vi "Write To Log (append).vi"(8 "Error In":errorcluster, 11 "Text to write":string) -> (0 "Error Out":errorcluster)   [LabVIEW 2023, in "Error Manager.lvlib" / "Error Log.lvclass"]
uses:
  Error Log.lvclass
  Error Log Ref (class variable).vi
  Error Log.lvclass/Error Log.ctl
panel:
  # "Input\nInputs to the VI"
  # "Development\nControls or indicators that are useful for development or testing, but which are not outputs of the VI."
  # "Output\nOutputs of the VI"
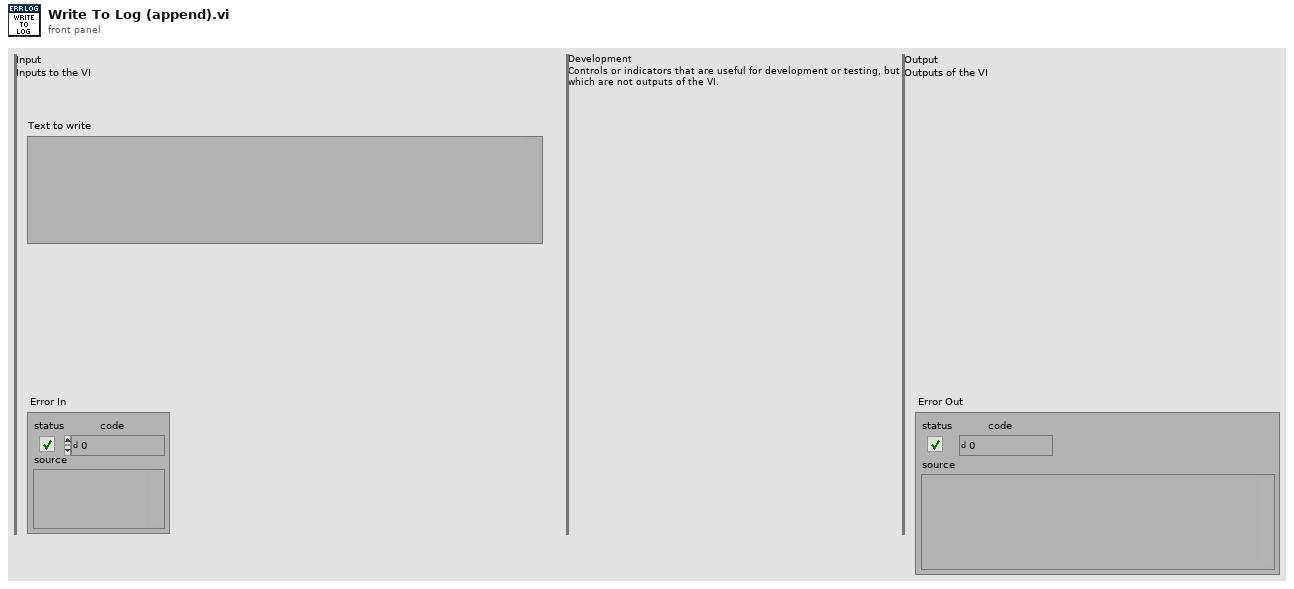
[diagram p1: front panel]
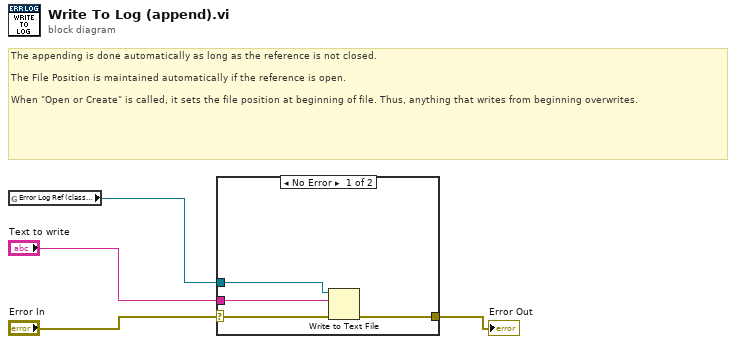
[diagram p0: block diagram]
diagram:
  # "The appending is done automatically as long as the reference is not closed.\n\nThe File Position is maintained automatically if the reference is open.\n\nWhen \"Open or Create\" is called, it sets the file position at beginning of file. Thus, anything that writes from beginning overwrites."
  n1 = global read "Error Log Ref (class variable).vi" item#0() -> (w2:refnum<file>)
  n2 = case shown="No Error" "Error In" {
    selector: "Error In" -> [w8 w9]
    tunnel: "Text to write" -> [w7 _]
    tunnel: w2 -> [w6 _]
    tunnel: [w5 w9] -> w1
    frame No Error {
      n3 = Write to Text File(file (use dialog)=w6, text=w7, error in=w8) -> (error out=w5:errorcluster)  [unwired: 1 in, 2 out]
    }
    frame Error {
    }
  }
  "Error Out" <- w1
